vi "DQMH_API_RunCreateEventDialog.vi"(8 "error in (no error)":errorcluster, 10 "Event":T1, 11 "ModuleName":string="TestStation.lvlib") -> (0 "error out":errorcluster, 3 "ViRef":refnum<vi>)   [LabVIEW 2016]
uses:
  <resource>/Framework/Providers/Open_GDS/UML/DQMH_API_class/EventCreationType.ctl
  <resource>/Framework/Providers/Open_GDS/UML/DQMHModuleNode_class/EventType.ctl
  <resource>/Framework/Providers/Open_GDS/UML/DQMHModuleNode_class/DQMHModuleNode.lvclass
  <resource>/Framework/Providers/Open_GDS/UML/DQMH_API_class/DQMH_API.lvclass
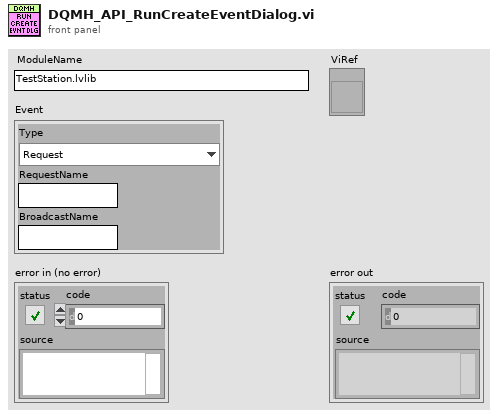
[diagram p1: front panel]
types:
  T1 = typedef "DQMH_API.lvclass/EventCreationType.ctl" = cluster{"Type":T2, "RequestName":string, "BroadcastName":string}
  T2 = typedef "DQMHModuleNode.lvclass/EventType.ctl" = enum16{"Request", "Request and Wait For Reply", "Roundtrip", "Broadcast"}
  T3 = cluster{"Cancelled":bool, "ViRef":refnum<vi>, "ControlValues":refnum<vi>[]}
  T4 = enum32{"Bad", "Idle", "Run top level", "Running"}
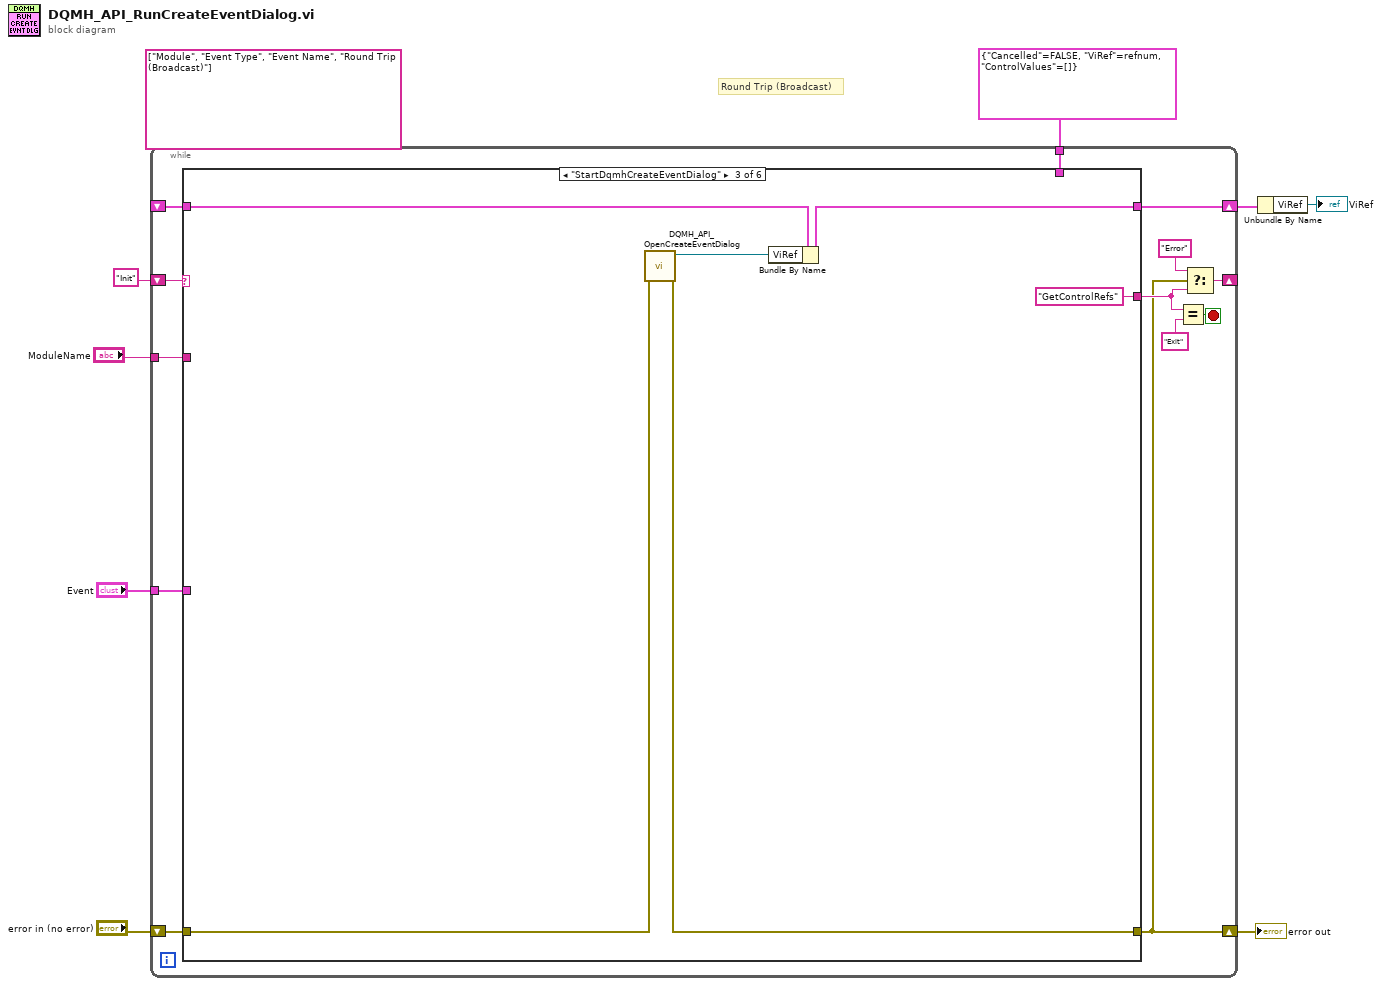
[diagram p0: block diagram]
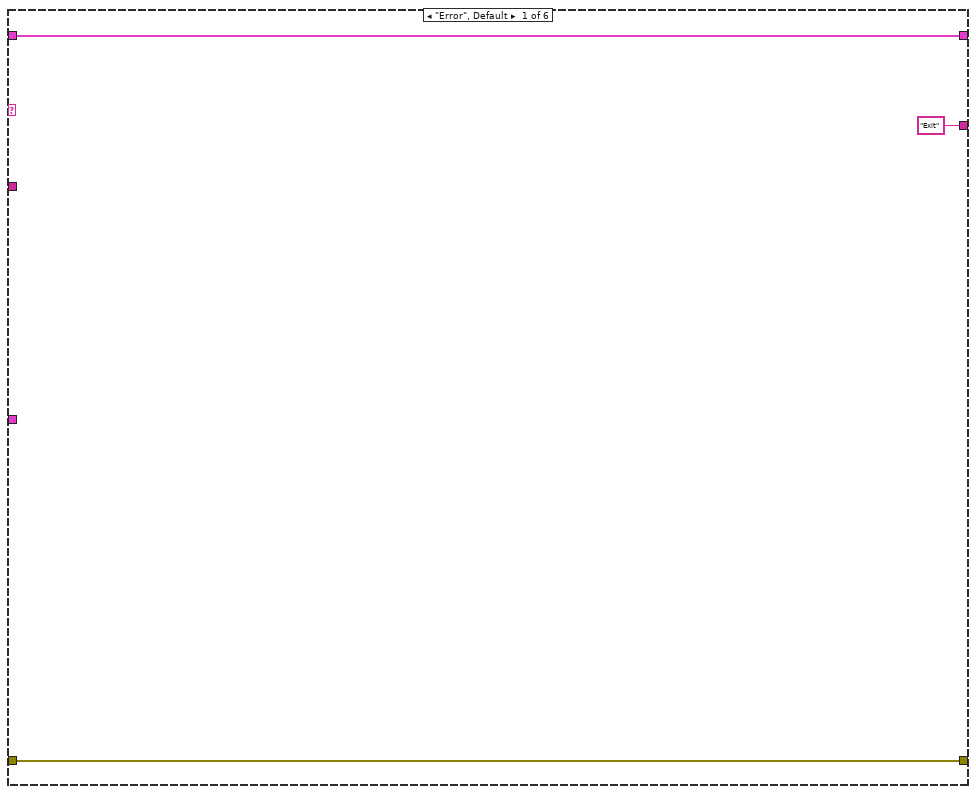
[diagram p2: hidden frame]
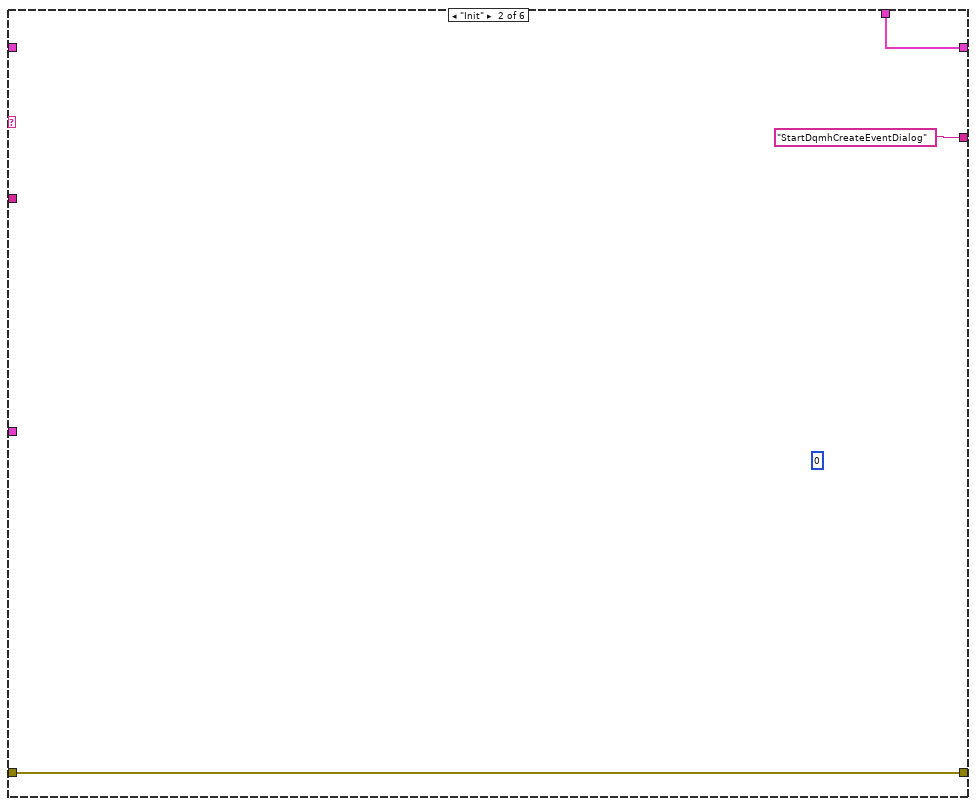
[diagram p3: hidden frame]
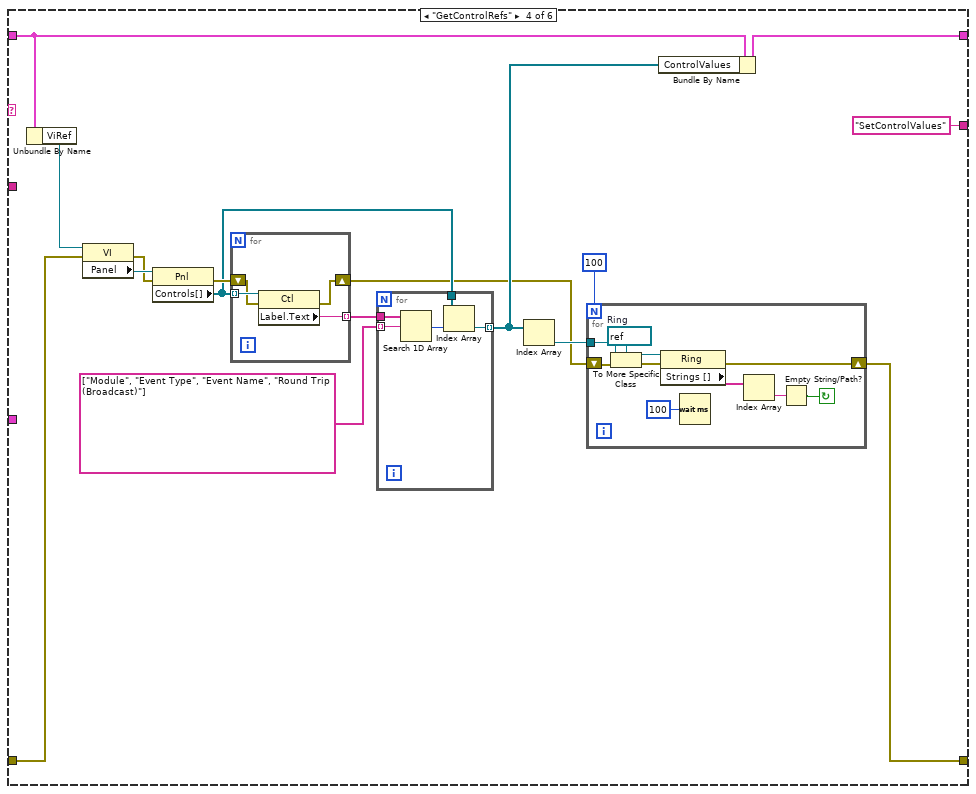
[diagram p4: hidden frame]
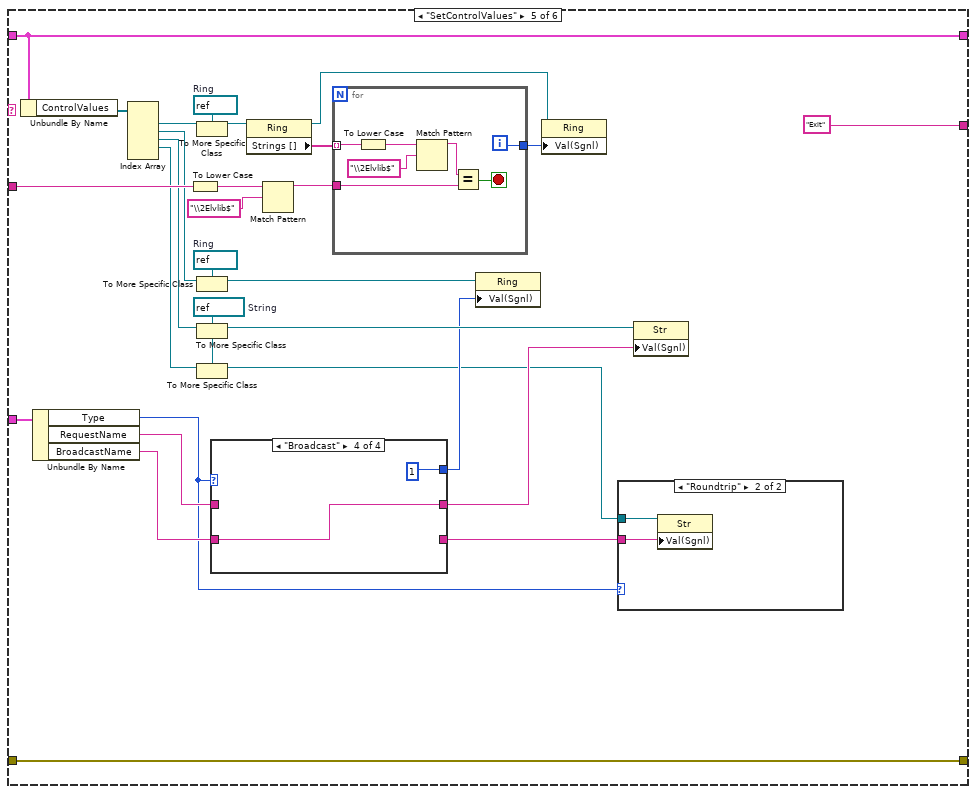
[diagram p5: hidden frame]
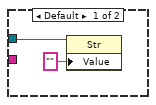
[diagram p6: hidden frame]
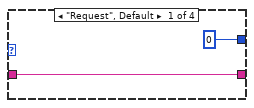
[diagram p7: hidden frame]
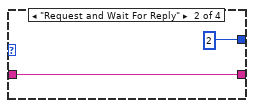
[diagram p8: hidden frame]
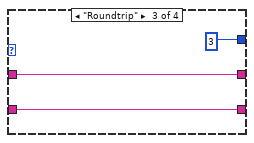
[diagram p9: hidden frame]
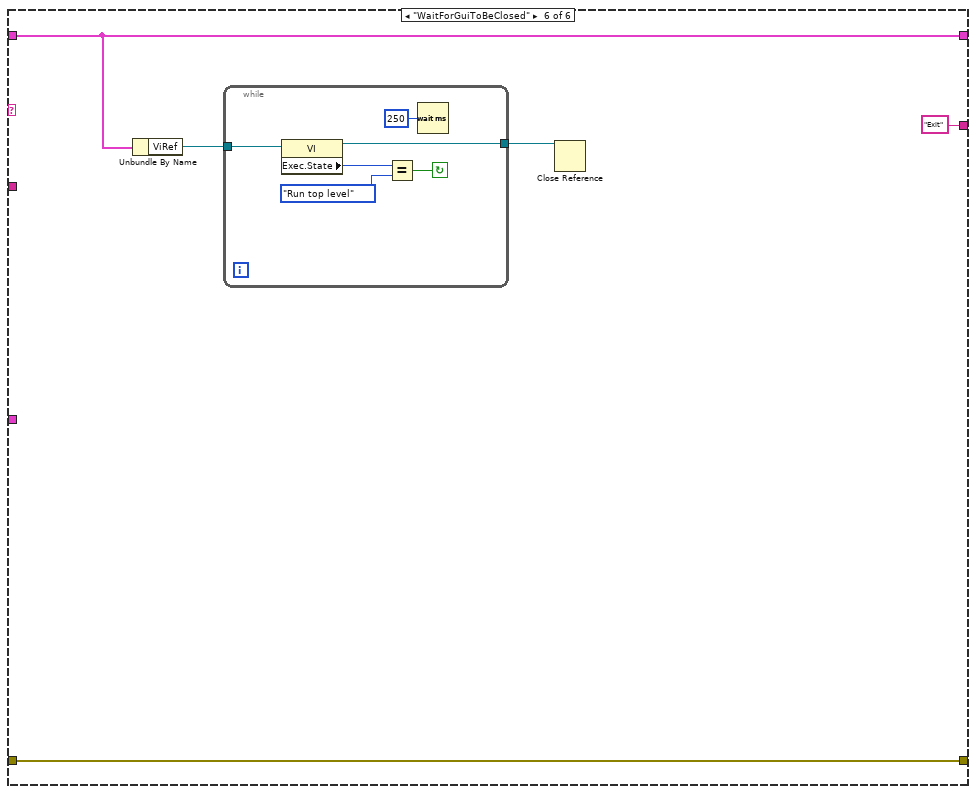
[diagram p10: hidden frame]
diagram:
  (unwired) string[] ["Module", "Event Type", "Event Name", "Round Trip (Broadcast)"]
  # "Round Trip (Broadcast)"
  n1 = while {
    shift-right: [w14] -> w5
    shift-left: "error in (no error)" -> [w21]
    shift-right: [w19] -> _
    shift-left: "Init" -> [w20]
    shift-right: [w13] -> w8
    shift-left: _ -> [w12]
    tunnel: T3 {"Cancelled"=FALSE, "ViRef"=refnum, "ControlValues"=[]} -> [w11]
    tunnel: "ModuleName" -> [w10]
    tunnel: "Event" -> [w9]
    stop <- w18 stop-if-true
    n2 = case shown="\"StartDqmhCreateEventDialog\"" w20 {
      tunnel: w21 -> [w24 w26 w29 w46 w97 w118]
      tunnel: [w24 w26 w28 w36 w97 w118] -> w14
      tunnel: ["Exit" "StartDqmhCreateEventDialog" "GetControlRefs" "SetControlValues" "Exit" "Exit"] -> w15
      tunnel: [w22 w25 w31 w38 w95 w122] -> w13
      tunnel: w12 -> [w22 _ w32 w48 w95 w122]
      tunnel: w11 -> [_ w25 _ _ _ _]
      tunnel: w10 -> [_ _ _ _ w87 _]
      tunnel: w9 -> [_ _ _ _ w83 _]
      frame "Error", Default {
      }
      frame "Init" {
        (unwired) 0 ("Counter")
      }
      frame "StartDqmhCreateEventDialog" {
        n3 = call <resource>:"DQMH_API_OpenCreateEventDialog.vi"("error in (no error)"=w29) -> ("error out"=w28:errorcluster, "DqmhCreateEventDialogRef"=w30:refnum<vi>)  [unwired: 8 in, 1 out]
        n4 = Bundle By Name(cluster=w32, "ViRef"=w30) -> (w31:T3)
      }
      frame "GetControlRefs" {
        n5 = Unbundle By Name(w48) -> ("ViRef"=w47:refnum<vi>)
        n6 = property class="VI"(reference=w47, error in=w46) -> (error out=w45:errorcluster, "Panel"=w49:refnum<vi>)  [unwired: 1 out]
        n7 = property class="Pnl"(reference=w49, error in=w45) -> (error out=w44:errorcluster, "Controls[]"=w41:refnum<vi>[])  [unwired: 1 out]
        n8 = for {
          tunnel: w41 -> [w68] mode=indexing
          tunnel: [w67] -> w43 mode=indexing
          shift-right: [w65] -> w35
          shift-left: w44 -> [w66]
          n9 = property class="Ctl"(reference=w68, error in=w66) -> (error out=w65:errorcluster, "Label.Text"=w67:string)  [unwired: 1 out]
        }
        n10 = for {
          tunnel: w43 -> [w64]
          tunnel: string[] ["Module", "Event Type", "Event Name", "Round Trip (Broadcast)"] -> [w63] mode=indexing
          tunnel: w41 -> [w61]
          tunnel: [w60] -> w37 mode=indexing
          n11 = Search 1D Array(1D array=w64, element=w63) -> (index of element=w62:i32)  [unwired: 1 in]
          n12 = Index Array(array=w61, index=w62) -> (element=w60:refnum<vi>)
        }
        n13 = Index Array(array=w37) -> (element=w40:refnum<vi>)  [unwired: 1 in]
        n14 = for {
          N: 100 -> [_]
          tunnel: w40 -> [w57]
          shift-right: [w52] -> w36
          shift-left: w35 -> [w50]
          stop <- w53 continue-if-true
          w58 = refnum<vi> refnum  # Ring
          n15 = To More Specific Class(target class=w58, reference=w57, error in=w50) -> (specific class reference=w59:refnum<vi>, error out=w51:errorcluster)
          n16 = property class="Ring"(reference=w59, error in=w51) -> (error out=w52:errorcluster, "Strings []"=w55:string[])  [unwired: 1 out]
          n17 = Wait (ms)(milliseconds to wait=u32 100) -> ()  [unwired: 1 out]
          n18 = Index Array(array=w55) -> (element=w54:string)  [unwired: 1 in]
          n19 = Empty String/Path?(string/path=w54) -> (empty?=w53:bool)
        }
        n20 = Bundle By Name(cluster=w48, "ControlValues"=w37) -> (w38:T3)
      }
      frame "SetControlValues" {
        w78 = refnum<vi> refnum  # String
        w81 = refnum<vi> refnum  # Ring
        w91 = refnum<vi> refnum  # Ring
        n21 = Unbundle By Name(w95) -> ("ControlValues"=w94:refnum<vi>[])
        n22 = Unbundle By Name(w83) -> ("Type"=w69:T2, "RequestName"=w73:string, "BroadcastName"=w74:string)
        n23 = Index Array(array=w94) -> (element #1=w93:refnum<vi>, element #2=w82:refnum<vi>, element #3=w79:refnum<vi>, element #4=w77:refnum<vi>)  [unwired: 5 in, 1 out]
        n24 = To Lower Case(string=w87) -> (all lower case string=w88:string)
        n25 = To More Specific Class(target class=w91, reference=w93) -> (specific class reference=w92:refnum<vi>)  [unwired: 1 in, 1 out]
        n26 = To More Specific Class(target class=w81, reference=w82) -> (specific class reference=w80:refnum<vi>)  [unwired: 1 in, 1 out]
        n27 = To More Specific Class(target class=w78, reference=w79) -> (specific class reference=w76:refnum<vi>)  [unwired: 1 in, 1 out]
        n28 = To More Specific Class(target class=w78, reference=w77) -> (specific class reference=w70:refnum<vi>)  [unwired: 1 in, 1 out]
        n29 = case shown="\"Broadcast\"" w69 {
          tunnel: [0 2 3 1] -> w75
          tunnel: w74 -> [_ _ w106 w109]
          tunnel: [w102 w104 w107 w109] -> w72
          tunnel: w73 -> [w102 w104 w107 _]
          tunnel: [_ _ w106 _] -> w71
          frame "Request", Default {
          }
          frame "Request and Wait For Reply" {
          }
          frame "Roundtrip" {
          }
          frame "Broadcast" {
          }
        }
        n30 = property class="Ring"(reference=w92) -> (reference out=w85:refnum<vi>, "Strings []"=w90:string[])  [unwired: 1 in, 1 out]
        n31 = Match Pattern(string=w88, regular expression="\\2Elvlib$") -> (before substring=w86:string)  [unwired: 1 in, 3 out]
        n32 = for {
          tunnel: w90 -> [w117] mode=indexing
          tunnel: w86 -> [w113]
          tunnel: [w111] -> w84
          i -> [w111]
          stop <- w112 stop-if-true
          n33 = To Lower Case(string=w117) -> (all lower case string=w116:string)
          n34 = Match Pattern(string=w116, regular expression="\\2Elvlib$") -> (before substring=w114:string)  [unwired: 1 in, 3 out]
          n35 = Equal?(x=w114, y=w113) -> (x = y?=w112:bool)
        }
        n36 = property class="Ring"(reference=w80, "Val(Sgnl)"=w75) -> ()  [unwired: 1 in, 2 out]
        n37 = property class="Ring"(reference=w85, "Val(Sgnl)"=w84) -> ()  [unwired: 1 in, 2 out]
        n38 = case shown="\"Roundtrip\"" w69 {
          tunnel: w71 -> [_ w101]
          tunnel: w70 -> [w98 w100]
          frame Default {
            n39 = property class="Str"(reference=w98, "Value"="") -> ()  [unwired: 1 in, 2 out]
          }
          frame "Roundtrip" {
            n40 = property class="Str"(reference=w100, "Val(Sgnl)"=w101) -> ()  [unwired: 1 in, 2 out]
          }
        }
        n41 = property class="Str"(reference=w76, "Val(Sgnl)"=w72) -> ()  [unwired: 1 in, 2 out]
      }
      frame "WaitForGuiToBeClosed" {
        n42 = Unbundle By Name(w122) -> ("ViRef"=w121:refnum<vi>)
        n43 = while {
          tunnel: w121 -> [w128]
          tunnel: [w123] -> w120
          stop <- w125 continue-if-true
          n44 = property class="VI"(reference=w128) -> (reference out=w123:refnum<vi>, "Exec.State"=w127:T4)  [unwired: 1 in, 1 out]
          n45 = Equal?(x=w127, y=T4."Run top level") -> (x = y?=w125:bool)
          n46 = Wait (ms)(milliseconds to wait=u32 250) -> ()  [unwired: 1 out]
        }
        n47 = Close Reference(reference=w120) -> ()  [unwired: 1 in, 1 out]
      }
    }
    n48 = Equal?(x=w15, y="Exit") -> (x = y?=w18:bool)
    n49 = Select(t="Error", s=w14, f=w15) -> (s? t:f=w19:string)
  }
  "error out" <- w5
  n50 = Unbundle By Name(w8) -> ("ViRef"=→"ViRef":refnum<vi>)
